vi "ROI group-Event handler-Groups array value change.vi"(9 "OldVal":T1[](array[typedef]), 10 "NewVal":T1[](array[typedef]), 11 "[Groups]":T2) -> ()   [LabVIEW 2020]
uses:
  Typedefs/Groups array referecne.ctl
  Typedefs/Group sel cluster.ctl
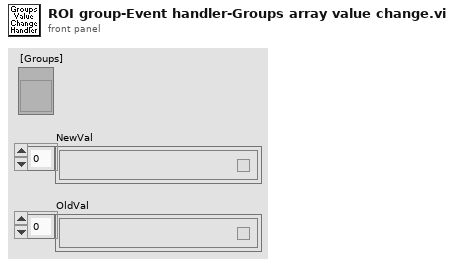
[diagram p1: front panel]
types:
  T1 = typedef "Group sel cluster.ctl" = cluster{"Group number":string, "Group Name":string, "Visibility":bool, "Highlight":bool}
  T2 = typedef "Groups array referecne.ctl" = refnum<vi>
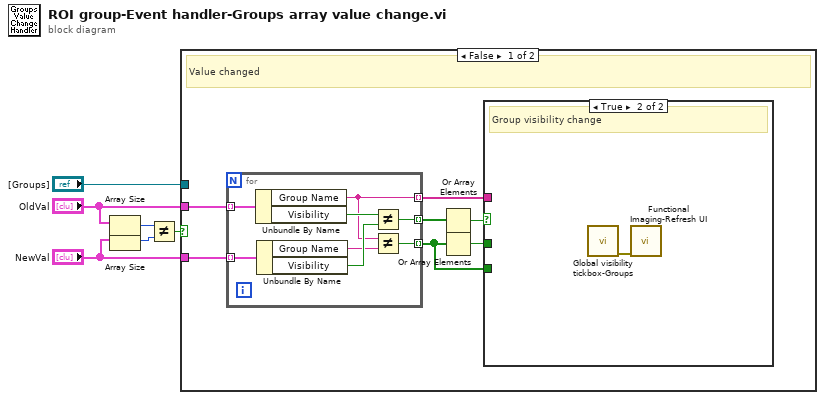
[diagram p0: block diagram]
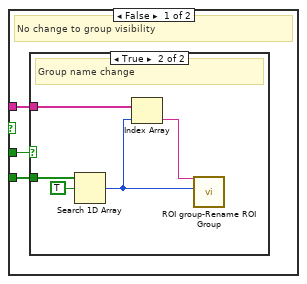
[diagram p2: hidden frame]
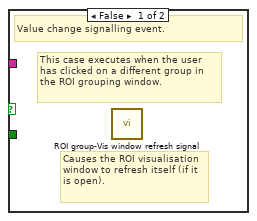
[diagram p3: hidden frame]
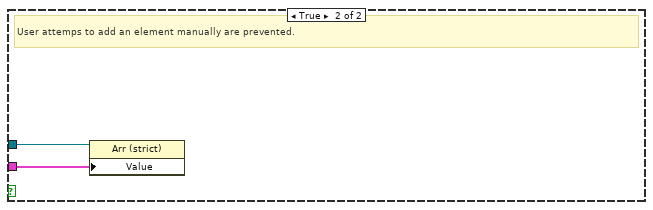
[diagram p4: hidden frame]
diagram:
  n1 = Array Size(array="OldVal") -> (size(s)=w3:i32)
  n2 = Array Size(array="NewVal") -> (size(s)=w4:i32)
  n3 = Not Equal?(x=w3, y=w4) -> (x != y?=w5:bool)
  n4 = case shown="False" w5 {
    tunnel: "OldVal" -> [w13 w32]
    tunnel: "[Groups]" -> [_ w31]
    tunnel: "NewVal" -> [w12 _]
    frame False {
      # "Value changed"
      n5 = for {
        tunnel: w13 -> [w30] mode=indexing
        tunnel: w12 -> [w29] mode=indexing
        tunnel: [w25] -> w11 mode=indexing
        tunnel: [w24] -> w8 mode=indexing
        tunnel: [w23] -> w7 mode=indexing
        n6 = Unbundle By Name(w30) -> ("Group Name"=w23:string, "Visibility"=w28:bool)
        n7 = Unbundle By Name(w29) -> ("Group Name"=w26:string, "Visibility"=w27:bool)
        n8 = Not Equal?(x=w28, y=w27) -> (x != y?=w25:bool)
        n9 = Not Equal?(x=w23, y=w26) -> (x != y?=w24:bool)
      }
      n10 = Or Array Elements(Boolean array=w11) -> (logical OR=w10:bool)
      n11 = Or Array Elements(Boolean array=w8) -> (logical OR=w9:bool)
      n12 = case shown="True" w10 {
        tunnel: w9 -> [w16 _]
        tunnel: w8 -> [w15 _]
        tunnel: w7 -> [w14 _]
        frame False {
          # "No change to group visibility"
          n13 = case shown="True" w16 {
            tunnel: w15 -> [_ w21]
            tunnel: w14 -> [_ w19]
            frame False {
              # "This case executes when the user\nhas clicked on a different group in\nthe ROI grouping window."
              # "Causes the ROI visualisation window to refresh itself (if it is open)."
              # "Value change signalling event."
              n14 = call "ROI group-Vis window refresh signal.vi"() -> ()  [unwired: 11 in, 1 out]
            }
            frame True {
              # "Group name change"
              n15 = Search 1D Array(1D array=w21, element=TRUE) -> (index of element=w18:i32)  [unwired: 1 in]
              n16 = Index Array(array=w19, index=w18) -> (element=w17:string)
              n17 = call "ROI group-Rename ROI Group.vi"("Index of renamed group"=w18, "Old group name"=w17) -> ()  [unwired: 9 in, 1 out]
            }
          }
        }
        frame True {
          # "Group visibility change"
          n18 = call "Global visibility tickbox-Groups.vi"() -> ("error out"=w22:errorcluster)  [unwired: 11 in]
          n19 = call "Functional Imaging-Refresh UI.vi"("error in (no error)"=w22) -> ()  [unwired: 11 in]
        }
      }
    }
    frame True {
      # "User attemps to add an element manually are prevented."
      n20 = property class="Arr (strict)"(reference=w31, "Value"=w32) -> ()  [unwired: 1 in, 2 out]
    }
  }
